vi "z keyexpr intersects.vi"(8 "error in (no error)":errorcluster, 10 "right":cluster{}, 11 "left":cluster{}) -> (0 "error out":errorcluster, 3 "function return":bool)   [LabVIEW 2021, in "zenohc.lvlib"]
doc: "bool z_keyexpr_intersects(const struct z_loaned_keyexpr_t *left,\n const struct z_loaned_keyexpr_t *right);"
uses:
  zenohc.lvlib
  zenohc.dll
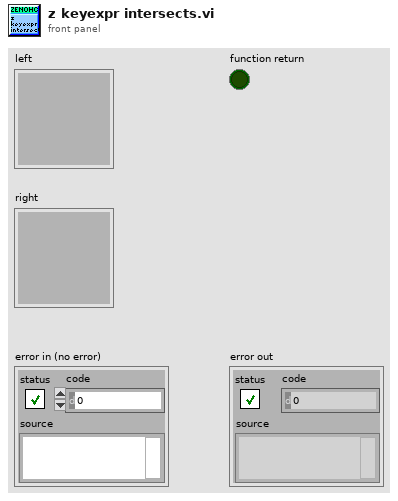
[diagram p1: front panel]
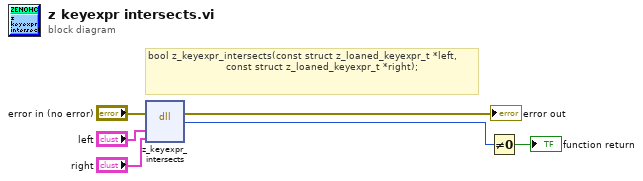
[diagram p0: block diagram]
diagram:
  # "bool z_keyexpr_intersects(const struct z_loaned_keyexpr_t *left,\n                          const struct z_loaned_keyexpr_t *right);"
  n1 = dll-call lib="D:/dev/zenoh_labview/zenohc/zenohc.*" fn="z_keyexpr_intersects"(error in="error in (no error)", "left"="left", "right"="right") -> (error out=→"error out":errorcluster, w5:u8)  [unwired: 4 in, 1 out]
  n2 = Not Equal To 0?(x=w5) -> (x != 0?=→"function return":bool)
